vi "Deploy to Device.vi"(8 "error in (no error)":errorcluster, 10 "Device":refnum<class "Device.lvclass">, 11 "AppDetailPanel in":refnum<class "AppDetailPanel.lvclass">) -> (0 "error out":errorcluster, 3 "AppDetailPanel out":refnum<class "AppDetailPanel.lvclass">)   [LabVIEW 2020, in "PicoG-App.lvlib" / "AppDetailPanel.lvclass"]
uses:
  AppDetailPanel.lvclass
  Device/Device.lvclass
  Deploy Data.ctl
  ViaApp/ViaApp.lvclass
  AppDetailPanel.lvclass/AppDetailPanel.ctl
  PicoG-App.lvlib
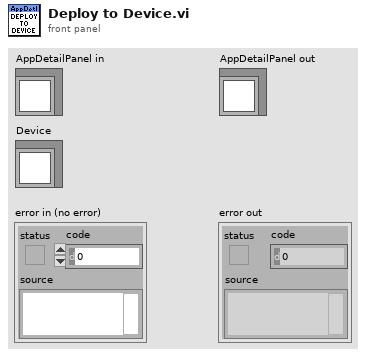
[diagram p1: front panel]
types:
  T1 = typedef "PicoG-App.lvlib/Deploy Data.ctl" = cluster{"App":refnum<class "ViaApp.lvclass">, "Device":refnum<class "Device.lvclass">}
  T2 = typedef "PicoG-App.lvlib/AppDetailPanel.lvclass/Ref Data.ctl" = cluster{"App":refnum<class "ViaApp.lvclass">}
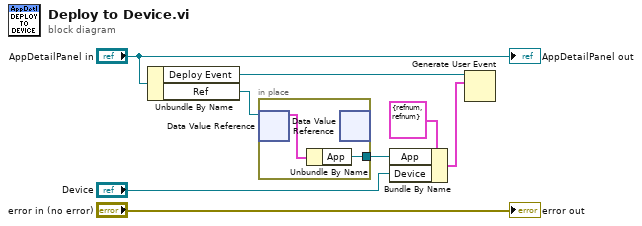
[diagram p0: block diagram]
diagram:
  n1 = Unbundle By Name("AppDetailPanel in") -> ("Deploy Event"=w2:refnum<user-event>, "Ref"=w7:refnum<data-value>)
  n2 = in-place {
    in-place-border: [w9] -> w4
    n3 = in-place-dvr #1(w7) -> (w10:T2)  [unwired: 1 out]
    n4 = Unbundle By Name(w10) -> ("App"=w9:refnum<class "ViaApp.lvclass">)
    n5 = in-place-dvr #1() -> ()  [unwired: 1 in, 2 out]
  }
  n6 = Bundle By Name(cluster=T1 {"App"=refnum, "Device"=refnum} ("Deploy Data"), "App"=w4, "Device"="Device") -> (w1:T1)
  n7 = Generate User Event(user event=w2, event data cluster=w1) -> ()  [unwired: 2 in, 2 out]
  "error out" <- "error in (no error)"
  "AppDetailPanel out" <- "AppDetailPanel in"
